vi "File - Save Controls to INI.vi"(7 "Section":string, 8 "error in (no error)":errorcluster, 9 "Array of References":refnum<vi>[](array[refnum]), 11 "INI File":path) -> (0 "error out":errorcluster)   [LabVIEW 2020]
doc: "Saves the values of a group of controls (passed as an array of references) to an INI file.\n\nThe control names are used for the key names (with spaces removed).\n\nWorks with digital/boolean/string/path/VISAResourceName and single level clusters."
uses:
  <vilib>/Utility/config.llb/Write Key (Double).vi
  <vilib>/Utility/config.llb/Write Key (U32).vi
  <vilib>/Utility/config.llb/Write Key (String).vi
  <vilib>/Utility/config.llb/NI_LVConfig.lvlib
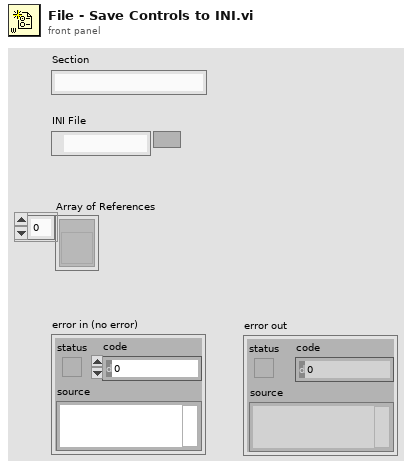
[diagram p1: front panel]
types:
  T1 = typedef "NI_LVConfig.lvlib/Config Data RefNum.ctl" = refnum<k1>
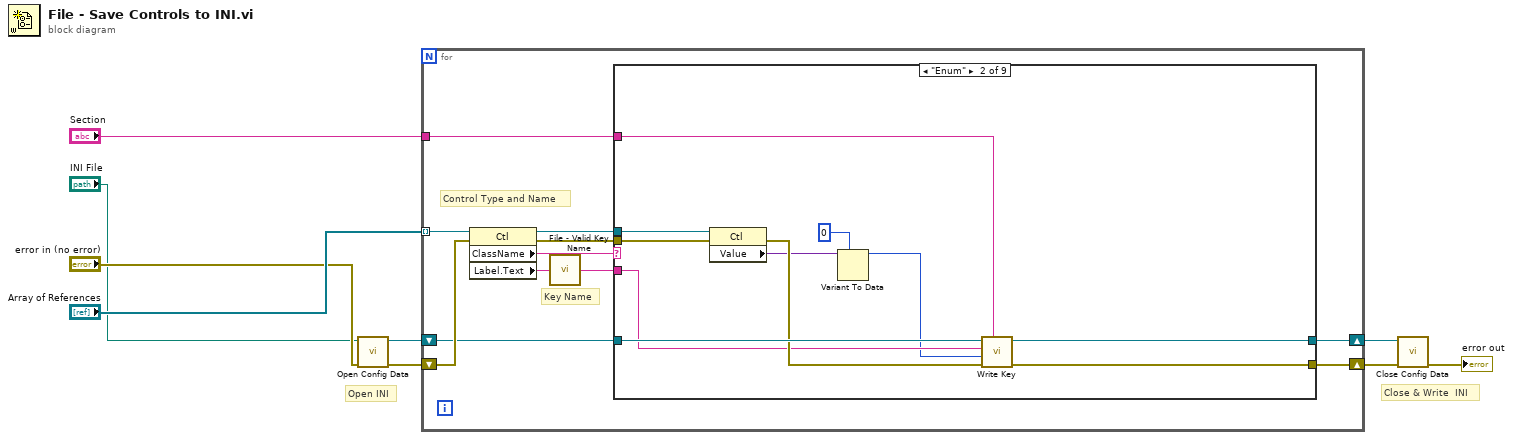
[diagram p0: block diagram]
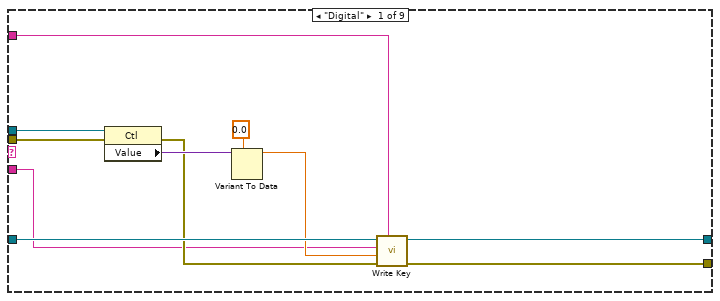
[diagram p2: hidden frame]
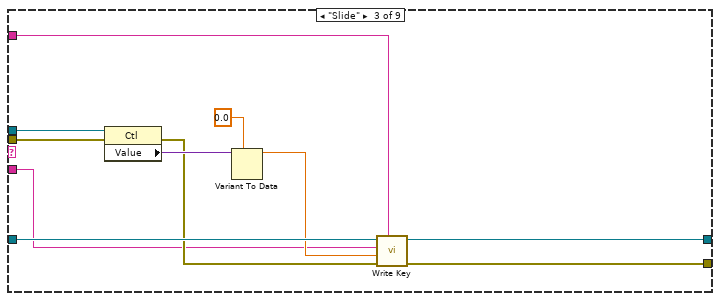
[diagram p3: hidden frame]
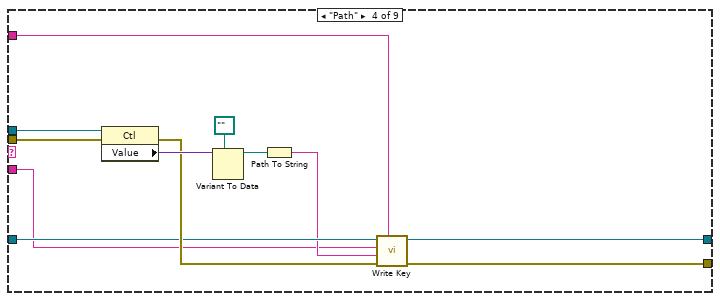
[diagram p4: hidden frame]
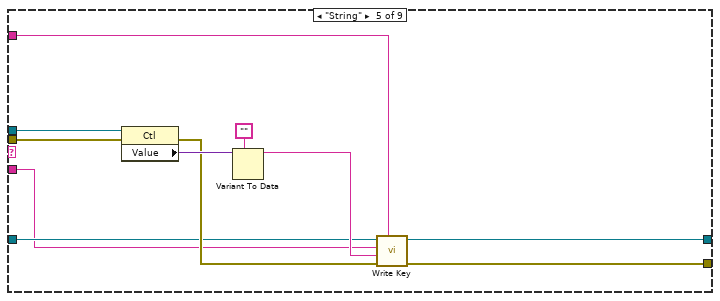
[diagram p5: hidden frame]
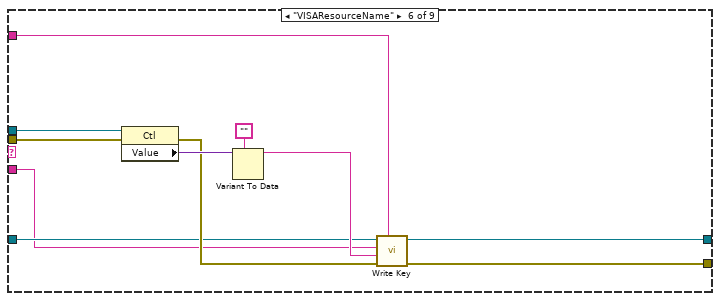
[diagram p6: hidden frame]
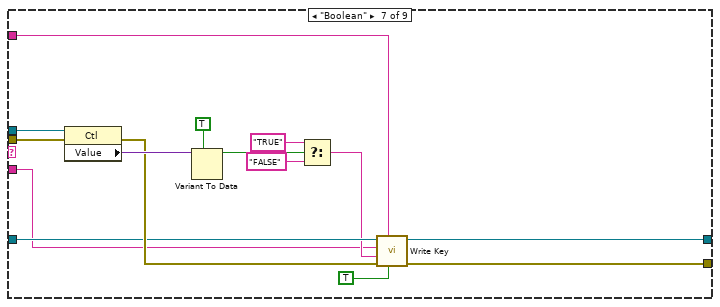
[diagram p7: hidden frame]
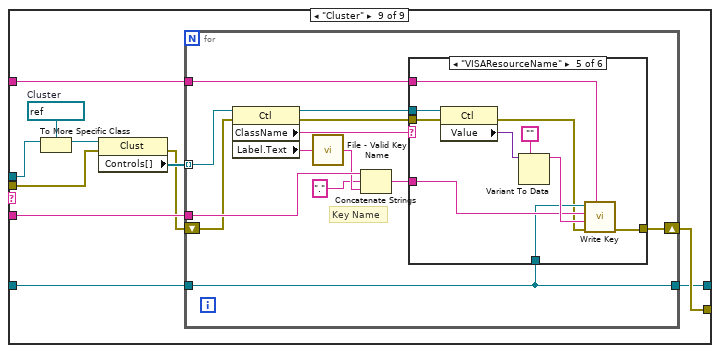
[diagram p9: hidden frame]
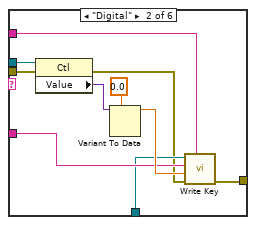
[diagram p11: hidden frame]
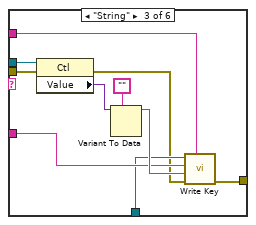
[diagram p12: hidden frame]
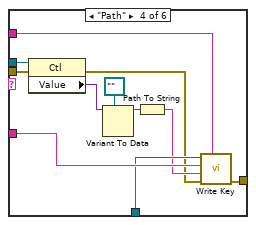
[diagram p13: hidden frame]
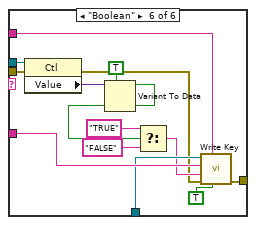
[diagram p14: hidden frame]
diagram:
  # "Close & Write  INI"
  # "Open INI"
  n1 = call <vilib>:"Open Config Data.vi"("error in (no error)"="error in (no error)", "configuration file path"="INI File") -> ("error out"=w5:errorcluster, "refnum"=w3:T1)  [unwired: 7 in, 1 out]
  n2 = for {
    tunnel: "Array of References" -> [w20] mode=indexing
    tunnel: "Section" -> [w17]
    shift-right: [w16] -> w7
    shift-left: w5 -> [w15]
    shift-right: [w13] -> w1
    shift-left: w3 -> [w12]
    # "Key Name"
    # "Control Type and Name"
    n3 = property class="Ctl"(reference=w20, error in=w15) -> (reference out=w18:refnum<vi>, error out=w14:errorcluster, "ClassName"=w19:string, "Label.Text"=w11:string)
    n4 = call "File - Valid Key Name.vi"("Key Name In"=w11) -> ("Key Name Out"=w10:string)  [unwired: 4 in]
    n5 = case shown="\"Enum\"" w19 {
      tunnel: w18 -> [w31 w42 w53 w65 w76 w87 w102 _ w115]
      tunnel: w10 -> [w21 w36 w44 w54 w66 w77 w88 _ w110]
      tunnel: w17 -> [w27 w35 w50 w61 w72 w83 w95 _ w108]
      tunnel: w14 -> [w28 w41 w51 w62 w73 w84 w96 w104 w111]
      tunnel: [w24 w38 w47 w60 w71 w82 w94 w104 w109] -> w16
      tunnel: [w25 w39 w48 w57 w68 w79 w92 w103 w106] -> w13
      tunnel: w12 -> [w26 w40 w49 w58 w67 w78 w91 w103 w107]
      frame "Digital" {
        n6 = property class="Ctl"(reference=w31, error in=w28) -> (error out=w23:errorcluster, "Value"=w30:variant)  [unwired: 1 out]
        n7 = Variant To Data(type=0.0 ("Total"), Variant=w30) -> (data=w22:dbl)  [unwired: 1 in, 1 out]
        n8 = call-poly <vilib>:"Write Key.vi"("section"=w27, "error in (no error)"=w23, "value"=w22, "key"=w21, "refnum"=w26) -> ("error out"=w24:errorcluster, "refnum out"=w25:T1)  [unwired: 4 in, 1 out]
      }
      frame "Enum" {
        n9 = property class="Ctl"(reference=w42, error in=w41) -> (error out=w37:errorcluster, "Value"=w33:variant)  [unwired: 1 out]
        n10 = Variant To Data(type=u16 0 ("unsigned 16bit integer"), Variant=w33) -> (data=w32:u16)  [unwired: 1 in, 1 out]
        n11 = call-poly <vilib>:"Write Key.vi"("section"=w35, "error in (no error)"=w37, "value"=w32, "key"=w36, "refnum"=w40) -> ("error out"=w38:errorcluster, "refnum out"=w39:T1)  [unwired: 4 in, 1 out]
      }
      frame "Slide" {
        n12 = property class="Ctl"(reference=w53, error in=w51) -> (error out=w46:errorcluster, "Value"=w52:variant)  [unwired: 1 out]
        n13 = Variant To Data(type=0.0, Variant=w52) -> (data=w45:dbl)  [unwired: 1 in, 1 out]
        n14 = call-poly <vilib>:"Write Key.vi"("section"=w50, "error in (no error)"=w46, "value"=w45, "key"=w44, "refnum"=w49) -> ("error out"=w47:errorcluster, "refnum out"=w48:T1)  [unwired: 4 in, 1 out]
      }
      frame "Path" {
        n15 = property class="Ctl"(reference=w65, error in=w62) -> (error out=w59:errorcluster, "Value"=w64:variant)  [unwired: 1 out]
        n16 = Variant To Data(type=path "", Variant=w64) -> (data=w56:path)  [unwired: 1 in, 1 out]
        n17 = Path To String(path=w56) -> (string=w55:string)
        n18 = call-poly <vilib>:"Write Key.vi"("section"=w61, "error in (no error)"=w59, "value"=w55, "key"=w54, "refnum"=w58) -> ("error out"=w60:errorcluster, "refnum out"=w57:T1)  [unwired: 4 in, 1 out]
      }
      frame "String" {
        n19 = property class="Ctl"(reference=w76, error in=w73) -> (error out=w70:errorcluster, "Value"=w75:variant)  [unwired: 1 out]
        n20 = Variant To Data(type="", Variant=w75) -> (data=w69:string)  [unwired: 1 in, 1 out]
        n21 = call-poly <vilib>:"Write Key.vi"("section"=w72, "error in (no error)"=w70, "value"=w69, "key"=w66, "refnum"=w67) -> ("error out"=w71:errorcluster, "refnum out"=w68:T1)  [unwired: 4 in, 1 out]
      }
      frame "VISAResourceName" {
        n22 = property class="Ctl"(reference=w87, error in=w84) -> (error out=w81:errorcluster, "Value"=w86:variant)  [unwired: 1 out]
        n23 = Variant To Data(type="", Variant=w86) -> (data=w80:string)  [unwired: 1 in, 1 out]
        n24 = call-poly <vilib>:"Write Key.vi"("section"=w83, "error in (no error)"=w81, "value"=w80, "key"=w77, "refnum"=w78) -> ("error out"=w82:errorcluster, "refnum out"=w79:T1)  [unwired: 4 in, 1 out]
      }
      frame "Boolean" {
        n25 = property class="Ctl"(reference=w102, error in=w96) -> (error out=w93:errorcluster, "Value"=w101:variant)  [unwired: 1 out]
        n26 = Variant To Data(type=TRUE, Variant=w101) -> (data=w99:bool)  [unwired: 1 in, 1 out]
        n27 = Select(t="TRUE", s=w99, f="FALSE") -> (s? t:f=w90:string)
        n28 = call-poly <vilib>:"Write Key.vi"("write raw string? (F)"=TRUE, "section"=w95, "error in (no error)"=w93, "value"=w90, "key"=w88, "refnum"=w91) -> ("error out"=w94:errorcluster, "refnum out"=w92:T1)  [unwired: 3 in, 1 out]
      }
      frame Default {
      }
      frame "Cluster" {
        w113 = refnum<vi> refnum  # Cluster
        n29 = To More Specific Class(target class=w113, reference=w115) -> (specific class reference=w114:refnum<vi>)  [unwired: 1 in, 1 out]
        n30 = property class="Clust"(reference=w114, error in=w111) -> (error out=w105:errorcluster, "Controls[]"=w112:refnum<vi>[])  [unwired: 1 out]
        n31 = for {
          tunnel: w112 -> [w128] mode=indexing
          tunnel: w110 -> [w126]
          shift-right: [w122] -> w109
          shift-left: w105 -> [w118]
          tunnel: w108 -> [w120]
          tunnel: w107 -> [w119]
          tunnel: [w119] -> w106
          # "Key Name"
          n32 = property class="Ctl"(reference=w128, error in=w118) -> (reference out=w121:refnum<vi>, error out=w117:errorcluster, "ClassName"=w116:string, "Label.Text"=w127:string)
          n33 = call "File - Valid Key Name.vi"("Key Name In"=w127) -> ("Key Name Out"=w125:string)  [unwired: 4 in]
          n34 = Concatenate Strings(w126, ".", w125) -> (w123:string)
          n35 = case shown="\"VISAResourceName\"" w116 {
            tunnel: w123 -> [_ w133 w143 w154 w164 w179]
            tunnel: [w129 w136 w146 w157 w167 w181] -> w122
            tunnel: w121 -> [_ w139 w149 w160 w170 w184]
            tunnel: w120 -> [_ w135 w145 w156 w166 w180]
            tunnel: w119 -> [_ w132 w142 w153 w163 w178]
            tunnel: w117 -> [w129 w131 w141 w151 w162 w172]
            frame Default {
            }
            frame "Digital" {
              n36 = property class="Ctl"(reference=w139, error in=w131) -> (error out=w130:errorcluster, "Value"=w137:variant)  [unwired: 1 out]
              n37 = Variant To Data(type=0.0 ("Total"), Variant=w137) -> (data=w134:dbl)  [unwired: 1 in, 1 out]
              n38 = call-poly <vilib>:"Write Key.vi"("section"=w135, "error in (no error)"=w130, "value"=w134, "key"=w133, "refnum"=w132) -> ("error out"=w136:errorcluster)  [unwired: 4 in, 2 out]
            }
            frame "String" {
              n39 = property class="Ctl"(reference=w149, error in=w141) -> (error out=w140:errorcluster, "Value"=w147:variant)  [unwired: 1 out]
              n40 = Variant To Data(type="" ("Total"), Variant=w147) -> (data=w144:string)  [unwired: 1 in, 1 out]
              n41 = call-poly <vilib>:"Write Key.vi"("section"=w145, "error in (no error)"=w140, "value"=w144, "key"=w143, "refnum"=w142) -> ("error out"=w146:errorcluster)  [unwired: 4 in, 2 out]
            }
            frame "Path" {
              n42 = property class="Ctl"(reference=w160, error in=w151) -> (error out=w150:errorcluster, "Value"=w158:variant)  [unwired: 1 out]
              n43 = Variant To Data(type=path "" ("Total"), Variant=w158) -> (data=w155:path)  [unwired: 1 in, 1 out]
              n44 = Path To String(path=w155) -> (string=w152:string)
              n45 = call-poly <vilib>:"Write Key.vi"("section"=w156, "error in (no error)"=w150, "value"=w152, "key"=w154, "refnum"=w153) -> ("error out"=w157:errorcluster)  [unwired: 4 in, 2 out]
            }
            frame "VISAResourceName" {
              n46 = property class="Ctl"(reference=w170, error in=w162) -> (error out=w161:errorcluster, "Value"=w168:variant)  [unwired: 1 out]
              n47 = Variant To Data(type="" ("Total"), Variant=w168) -> (data=w165:string)  [unwired: 1 in, 1 out]
              n48 = call-poly <vilib>:"Write Key.vi"("section"=w166, "error in (no error)"=w161, "value"=w165, "key"=w164, "refnum"=w163) -> ("error out"=w167:errorcluster)  [unwired: 4 in, 2 out]
            }
            frame "Boolean" {
              n49 = property class="Ctl"(reference=w184, error in=w172) -> (error out=w171:errorcluster, "Value"=w182:variant)  [unwired: 1 out]
              n50 = Variant To Data(type=TRUE, Variant=w182) -> (data=w175:bool)  [unwired: 1 in, 1 out]
              n51 = Select(t="TRUE", s=w175, f="FALSE") -> (s? t:f=w174:string)
              n52 = call-poly <vilib>:"Write Key.vi"("write raw string? (F)"=TRUE, "section"=w180, "error in (no error)"=w171, "value"=w174, "key"=w179, "refnum"=w178) -> ("error out"=w181:errorcluster)  [unwired: 3 in, 2 out]
            }
          }
        }
      }
    }
  }
  n53 = call <vilib>:"Close Config Data.vi"("error in (no error)"=w7, "refnum"=w1) -> ("error out"=→"error out":errorcluster)  [unwired: 8 in, 1 out]
